vi "SetGXMLCfgCurrent.vi"(8 "error in (no error)":errorcluster, 10 "CurrentChanCfg":T1, 11 "Current in":refnum<class "Current.lvclass">) -> (0 "error out":errorcluster, 3 "Current out":refnum<class "Current.lvclass">)   [LabVIEW 2018, in "Measurement Channels.lvlib" / "Current.lvclass"]
uses:
  Current.lvclass
  CurrentProps_TD.ctl
  Current.lvclass/Current.ctl
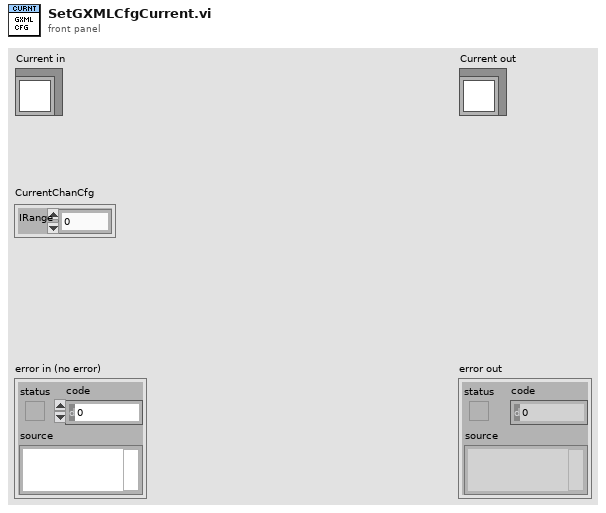
[diagram p1: front panel]
types:
  T1 = typedef "CurrentProps_TD.ctl" = cluster{"IRange":dbl}
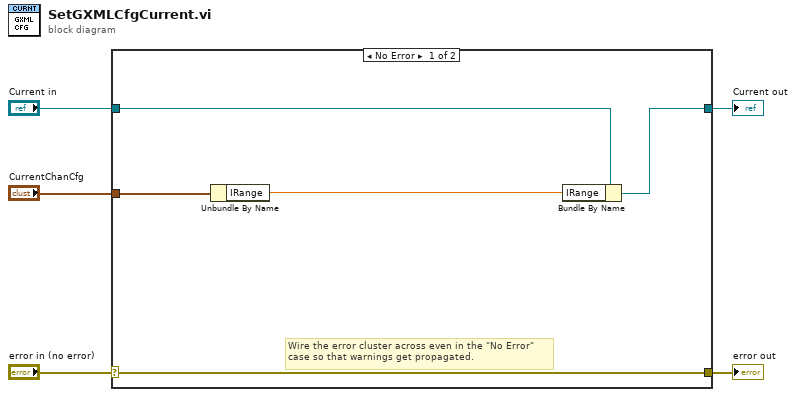
[diagram p0: block diagram]
diagram:
  n1 = case shown="No Error" "error in (no error)" {
    selector: "error in (no error)" -> [w10 w12]
    tunnel: [w10 w12] -> w4
    tunnel: [w7 w11] -> w2
    tunnel: "Current in" -> [w8 w11]
    tunnel: "CurrentChanCfg" -> [w6 _]
    frame No Error {
      # "Wire the error cluster across even in the \"No Error\"\ncase so that warnings get propagated."
      n2 = Unbundle By Name(w6) -> ("IRange"=w9:dbl)
      n3 = Bundle By Name(cluster=w8, "IRange"=w9) -> (w7:refnum<class "Current.lvclass">)
    }
    frame Error {
    }
  }
  "error out" <- w4
  "Current out" <- w2
